vi "mainUI.vi"() -> ()   [LabVIEW 2017]
uses:
  globalUtilities.vi
panel:
  out "dropped frames":i32
  in  "acquisitionStart":bool
  in  "STOP":bool
  out "frame":u16[][](graph)
  in  "volume height (um)":dbl=80.0
  in  "volumes per second":dbl=3.0
  in  "GUI update divider":i32=16
  in  "frames per second":dbl=100.0
  out "folder name":string
  # "This VI sets all the acquisition parameters, starts the actual backend VI asynchronously, and displays the frames."
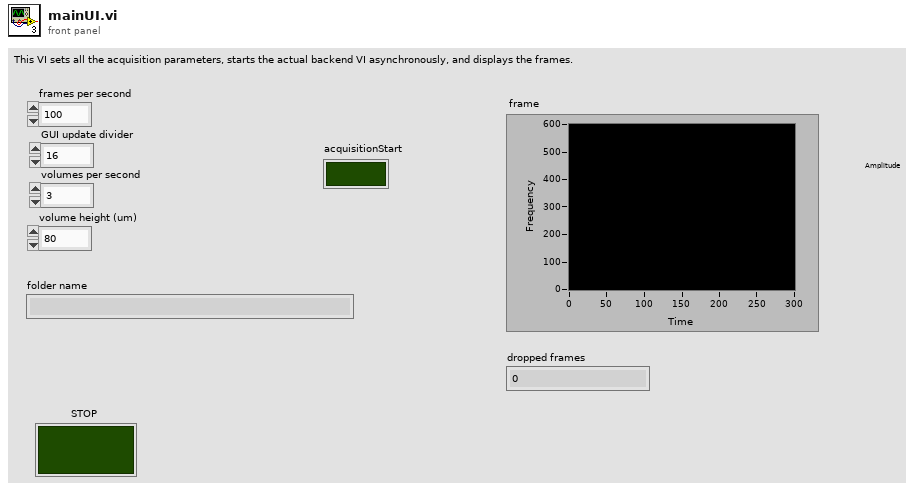
[diagram p1: front panel]
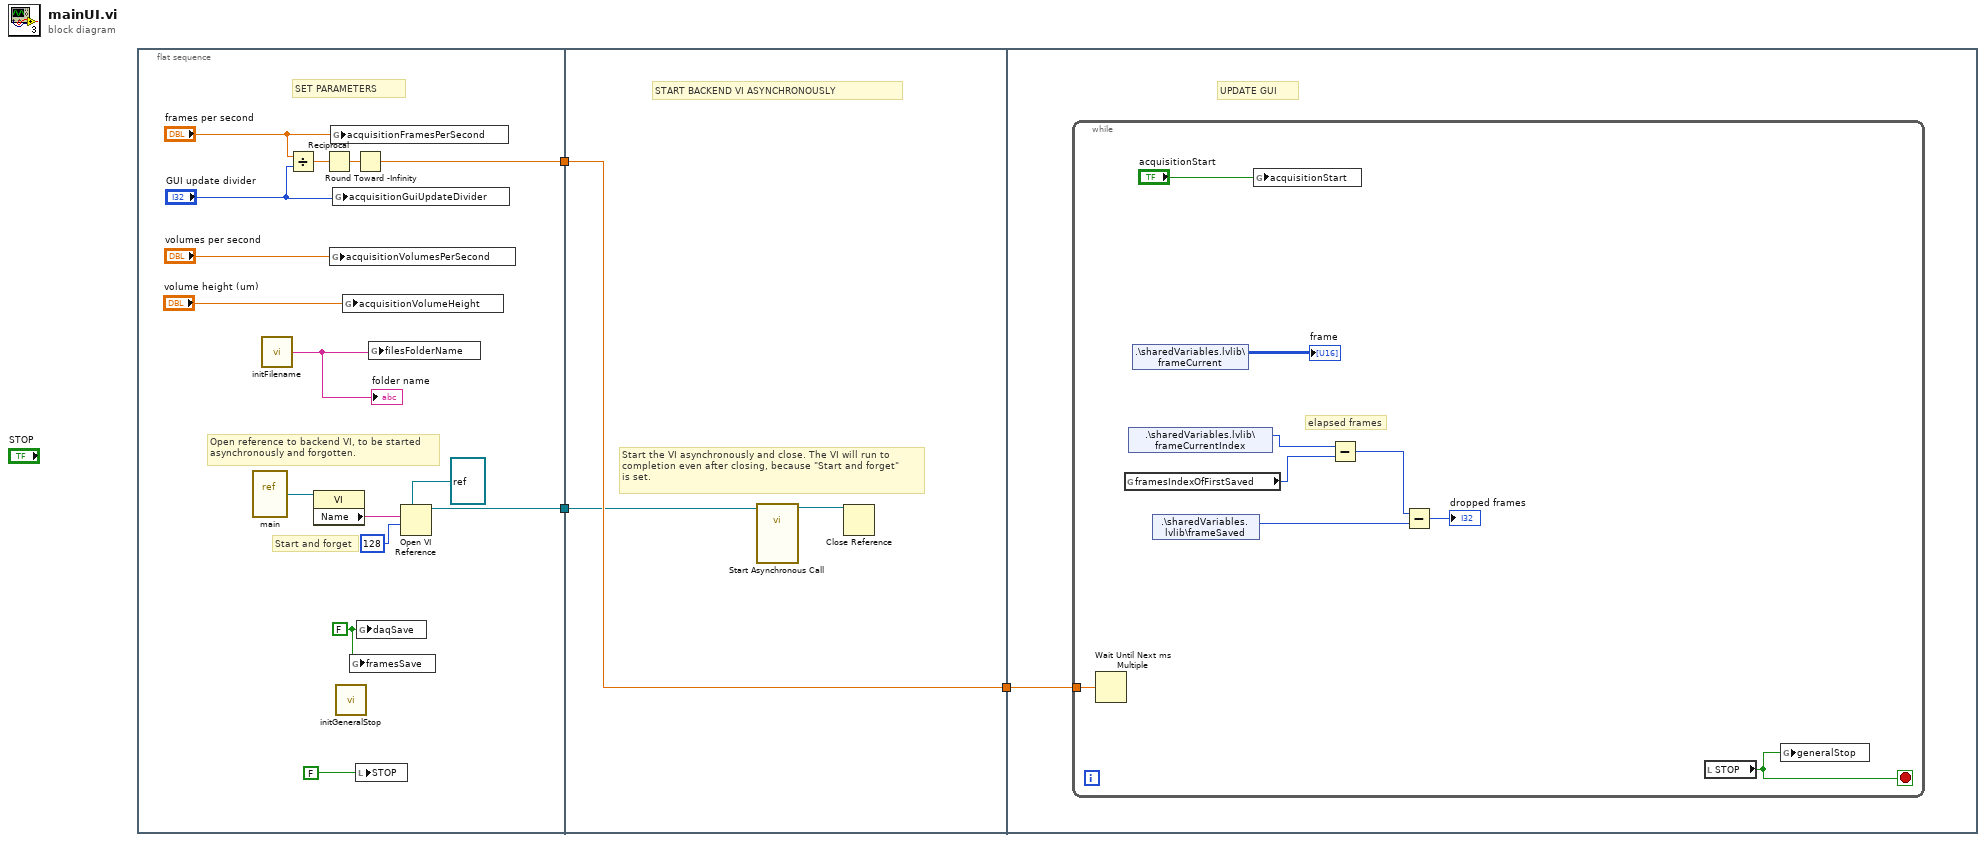
[diagram p0: block diagram]
diagram:
  n1 = flat-sequence {
    tunnel: [w11] -> w3
    tunnel: [w5] -> w1
    tunnel: w3 -> [w21]
    tunnel: [w21] -> w2
    tunnel: w1 -> [w20]
    tunnel: w2 -> [w22]
    frame #0 {
      w4 = FALSE ("daqSave")
      # "Start and forget"
      # "Open reference to backend VI, to be started\nasynchronously and forgotten."
      # "SET PARAMETERS"
      n2 = vi-ref "main.vi"() -> (w9:refnum<vi>)
      n3 = call "initFilename.vi"() -> ("folder name"=w18:string)  [unwired: 2 in]
      "folder name" <- w18
      n4 = Divide(x="frames per second", y="GUI update divider") -> (x/y=w13:dbl)
      n5 = property class="VI"(reference=w9) -> ("Name"=w8:string)  [unwired: 1 in, 2 out]
      n6 = Reciprocal(x=w13) -> (1/x=w12:dbl)
      n7 = global write "globalUtilities.vi" "acquisitionVolumesPerSecond"("volumes per second") -> ()
      n8 = global write "globalUtilities.vi" "acquisitionFramesPerSecond"("frames per second") -> ()
      n9 = global write "globalUtilities.vi" "acquisitionGuiUpdateDivider"("GUI update divider") -> ()
      n10 = call "initGeneralStop.vi"() -> ()  [unwired: 1 in]
      n11 = global write "globalUtilities.vi" "acquisitionVolumeHeight"("volume height (um)") -> ()
      n12 = global write "globalUtilities.vi" "framesSave"(w4) -> ()
      n13 = Round Toward -Infinity(1:w12) -> (0:w11:dbl)
      n14 = local write "STOP"(FALSE) -> ()
      n15 = global write "globalUtilities.vi" "daqSave"(w4) -> ()
      n16 = global write "globalUtilities.vi" "filesFolderName"(w18) -> ()
      n17 = Open VI Reference(type specifier VI Refnum (for type only)=refnum<vi> refnum, vi path=w8, options=128) -> (vi reference=w5:refnum<vi>)  [unwired: 3 in, 1 out]
    }
    frame #1 {
      # "Start the VI asynchronously and close. The VI will run to\ncompletion even after closing, because \"Start and forget\"\nis set."
      # "START BACKEND VI ASYNCHRONOUSLY"
      n18 = call-by-ref "Start Asynchronous Call"(reference=w20) -> (reference out=w19:refnum<vi>)  [unwired: 13 in, 1 out]
      n19 = Close Reference(reference=w19) -> ()  [unwired: 1 in, 1 out]
    }
    frame #2 {
      # "UPDATE GUI"
      n20 = while {
        tunnel: w22 -> [w31]
        stop <- w30 stop-if-true
        # "elapsed frames"
        n21 = Wait Until Next ms Multiple(millisecond multiple=w31) -> ()  [unwired: 1 out]
        n22 = global read "globalUtilities.vi" "framesIndexOfFirstSaved"() -> (w26:i32)
        n23 = shared-variable ".\\sharedVariables.lvlib\\frameCurrentIndex"() -> (w27:i32)  [unwired: 1 in, 1 out]
        n24 = shared-variable ".\\sharedVariables.lvlib\\frameCurrent"() -> (→"frame":u16[][])  [unwired: 1 in, 1 out]
        n25 = shared-variable ".\\sharedVariables.lvlib\\frameSaved"() -> (w24:u32)  [unwired: 1 in, 1 out]
        n26 = global write "globalUtilities.vi" "acquisitionStart"("acquisitionStart") -> ()
        n27 = Subtract(x=w27, y=w26) -> (x-y=w25:i32)
        n28 = Subtract(x=w25, y=w24) -> (x-y=→"dropped frames":u32)
        n29 = local read "STOP"() -> (w30:bool)
        n30 = global write "globalUtilities.vi" "generalStop"(w30) -> ()
      }
    }
  }
